vi "RandomLaser.vi"() -> ()   [LabVIEW 2014]
doc: "Random Laser Project\nAndré Romero - 2020\nandretec@ifsc.usp.br\n\nMain Program"
uses:
  OceanOptics.ctl
  PowerMeterSteps.ctl
  RL-Signal.ctl
  <vilib>/Analysis/2dsp.llb/Integral Method.ctl
  <vilib>/Analysis/8numeric.llb/1D Numeric Integration.vi
  GlobalVariables.vi
  <vilib>/Utility/file.llb/Write To Spreadsheet File (DBL).vi
  <vilib>/Analysis/NI_AAL_SigProc.lvlib
  <vilib>/Analysis/NI_AALBase.lvlib
  <vilib>/Analysis/NI_AALPro.lvlib
panel:
  in  "Stop":bool
  out "Power Meter":dbl[](array[numeric])=[-4.80034687e-05, -4.7408008e-05, -5.06443357e-05, -5.28425007e-05, -5.25678042e-05, -5.41400696e-05, -5.2216601e-05, -5.56666164e-05, -4.94078122e-05, -5.20333524e-05, -4.7408008e-05, -5.29950594e-05, -5.5727578e-05, -5.47354139e-05, -4.55456648e-05, -2.2403512e-05, -2.85706992e-05, -5.29950921e-05, -5.74067853e-05, -6.6779663e-05, -6.38182028e-05, -5.1773899e-05, -5.13617015e-05, -5.15602114e-05, -4.67210448e-05, -3.95311727e-05, -3.84473569e-05, -4.07676089e-05, -3.9119026e-05, -3.94700946e-05, -6.27801855e-05, -6.59400903e-05, -8.16175452e-05, -8.3525767e-05, -8.3525767e-05, -8.30677673e-05, -7.78622707e-05, -7.99309055e-06, 4.12680274e-05, 5.59075161e-05, 7.79505426e-05, 8.45298637e-05, 8.8880508e-05, 9.28800873e-05, 0.000106374602, 0.000115838942, 0.000191921004, 0.000232511724, 0.000233763392, 0.000173465407, 0.000158429335, 0.000152048175, 0.000145072074, 0.000134767964, 0.000126127823, 0.000116266419, 9.64061765e-05, 0.00010809963, 0.000134080954, 0.00013475267, 0.000128677129, 9.59789686e-05]
  out "Spectrum":dbl[][](array[numeric])
  out "Amplitudes":dbl[][](array[numeric])
  out "Locations Peaks":dbl[][](array[numeric])
  out "Integration":dbl[][](array[numeric])
  out "Integration":dbl[](array[numeric])
  out "size(s)":i32=105
  out "Waveform Graph 2":dbl[](graph)=[0.000604847446, 0.000604847446, 0.000604847446, 0.000688104541, 0.000688104541, 0.000688104541, 0.000688104541, 0.000915114302, 0.000915114302, 0.000915114302, 0.00125843158, 0.00125843158, 0.00125843158, 0.00169149181, 0.00169149181, 0.00169149181, 0.00169149181, 0.00235849386, 0.00235849386, 0.00235849386, 0.00235849386, 0.00314473268, 0.00314473268, 0.0041254824, 0.0041254824, 0.0041254824, 0.0041254824, 0.00483217463, 0.00483217463, 0.00483217463, 0.00559885986, 0.00559885986, 0.00559885986, 0.00559885986, 0.00666359905, 0.00666359905, 0.00666359905, 0.00792177953, 0.00792177953, 0.00792177953, 0.00792177953, 0.00900086574, 0.00900086574, 0.00900086574, 0.0102644078, 0.0102644078, 0.0102644078, 0.0102644078, 0.0114987111, 0.0114987111, 0.0114987111, 0.0114987111, 0.0129743796, 0.0129743796, 0.0129743796, 0.0141986832, 0.0141986832, 0.0141986832, 0.0141986832, 0.0155374203, 0.0155374203, 0.0155374203, 0.0155374203, 0.0168210845, 0.0168210845, 0.0168210845, 0.0182131026, 0.0182131026, 0.0182131026, 0.0182131026, 0.019541461, 0.019541461, 0.019541461, 0.0203341153, 0.0203341153, 0.0203341153, 0.0203341153, 0.0211376641, 0.0211376641, 0.0211376641, 0.0220639147, 0.0220639147, 0.0220639147, 0.0220639147, 0.0231049024, 0.0231049024, 0.0231049024, 0.0234890766, 0.0234890766, 0.0234890766, 0.0243229344, 0.0243229344, 0.0243229344, 0.0243229344, 0.0243483651, 0.0243483651, 0.0243483651, 0.0245883744, 0.0245883744, 0.0245883744, 0.0245883744, 0.0250559878, 0.0250559878, 0.0250559878, 0.0250559878]
  out "Motor Target":i32
  out "step error":dbl=5.243833813842798
  out "Numeric Control":i32=525
  out "appended array":dbl[](array[numeric])=[0.0239803754, 0.0238226056, 0.0238226056, 0.0238226056, 0.0243139379, 0.0243139379, 0.0243139379, 0.0243139379, 0.0240037385, 0.0240037385, 0.0240037385, 0.023470642, 0.023470642, 0.023470642, 0.0228483081, 0.0228483081, 0.0228483081, 0.0228483081, 0.0220416561, 0.0220416561, 0.0220416561, 0.0211109295, 0.0211109295, 0.0211109295, 0.0211109295, 0.0205111671, 0.0205111671, 0.0205111671, 0.0205111671, 0.0193525515, 0.0193525515, 0.0193525515, 0.0193525515, 0.0180644616, 0.0180644616, 0.0180644616, 0.0180644616, 0.0162604265, 0.0162604265, 0.0162604265, 0.0162604265, 0.015147699, 0.015147699, 0.0140616912, 0.0140616912, 0.0140616912, 0.0140616912, 0.0130754067, 0.0130754067, 0.0130754067, 0.0130754067, 0.0118028736, 0.0118028736, 0.0118028736, 0.0118028736, 0.00981818419, 0.00981818419, 0.00981818419, 0.00981818419, 0.00886647217, 0.00886647217, 0.00886647217, 0.00790723227, 0.00790723227, 0.00790723227, 0.00790723227, 0.00665996457, 0.00665996457, 0.00665996457, 0.00665996457, 0.00561416987, 0.00561416987, 0.00561416987, 0.00466312654, 0.00466312654, 0.00466312654, 0.00466312654, 0.00343694142, 0.00343694142, 0.00343694142, 0.00343694142, 0.00262781908, 0.00262781908, 0.00262781908, 0.00262781908, 0.00262781908, 0.0019172657, 0.0019172657, 0.0019172657, 0.0019172657, 0.0019172657, 0.00106541696, 0.00106541696, 0.00106541696, 0.00106541696, 0.000711521192, 0.000711521192, 0.000711521192, 0.000711521192, 0.000579979969, 0.000579979969, 0.000579979969, 0.000581125147, 0.000581125147, 0.000581125147, 0.000581125147, 0.000753699336, 0.000753699336, 0.000753699336, 0.000753699336, 0.00103271846, 0.00103271846, 0.00103271846, 0.00103271846, 0.00103271846, 0.00169448485, 0.00169448485, 0.00169448485, 0.00169448485, 0.00238372735, 0.00238372735, 0.00238372735, 0.00238372735, 0.00300710183, 0.00300710183, 0.00300710183, 0.00300710183, 0.00300710183, 0.00430094264, 0.00430094264, 0.00430094264, 0.00430094264, 0.00580574945, 0.00580574945, 0.00580574945, 0.00711680902, 0.00711680902, 0.00711680902, 0.00711680902, 0.0079354262, 0.0079354262, 0.0079354262, 0.0079354262, 0.00924165919, 0.00924165919, 0.00924165919, 0.0102110999, 0.0102110999, 0.0102110999, 0.0102110999, 0.0116844615, 0.0116844615, 0.0116844615, 0.0133227762, 0.0133227762, 0.0133227762, 0.0133227762, 0.0133227762, 0.0148326363, 0.0148326363, 0.0148326363, 0.0148326363, 0.0159355868, 0.0159355868, 0.0159355868, 0.0170806665, 0.0170806665, 0.0170806665, 0.0170806665, 0.0184924919, 0.0184924919, 0.0184924919, 0.0201629363, 0.0201629363, 0.0201629363, 0.0206157472, 0.0206157472, 0.0206157472, 0.0217395443, 0.0217395443, 0.0217395443, 0.0217395443, 0.0232210569, 0.0232210569, 0.0232210569, 0.023663858, 0.023663858, 0.023663858, 0.023663858, 0.023702329, 0.023702329, 0.023702329, 0.023702329, 0.0242230836, 0.0242230836, 0.0242230836, 0.0249410514, 0.0249410514, 0.0249410514, 0.0252798311, 0.0252798311, 0.0252798311, 0.0255696606, 0.0255696606, 0.0255696606, 0.0255696606, 0.0255696606, 0.025165854, 0.025165854, 0.025165854, 0.025165854, 0.0248792619, 0.0248792619, 0.0248792619, 0.0248792619, 0.0245558936, 0.0245558936, 0.0245558936, 0.0245558936, 0.024270013, 0.024270013, 0.024270013, 0.0235256515, 0.0235256515, 0.0235256515, 0.0235256515, 0.0228350237, 0.0228350237, 0.0228350237, 0.0228350237, 0.0225745663, 0.0225745663, 0.0225745663, 0.0225745663, 0.0210505258, 0.0210505258, 0.0210505258, 0.0210505258, 0.0199296717, 0.0199296717, 0.0199296717, 0.0199296717, 0.018528793, 0.018528793, 0.018528793, 0.018528793, 0.0175028276, 0.0175028276, 0.0175028276, 0.0158709381, 0.0158709381, 0.0158709381, 0.0158709381, 0.0138519667, 0.0138519667, 0.0138519667, 0.0131994681, 0.0131994681, 0.0131994681, 0.0131994681, 0.0117918346, 0.0117918346, 0.0117918346, 0.0107475519, 0.0107475519, 0.0107475519, 0.00919555873, 0.00919555873, 0.00919555873, 0.00919555873, 0.00811978336, 0.00811978336, 0.00811978336, 0.00811978336, 0.0069274581, 0.0069274581, 0.0069274581, 0.00582336541, 0.00582336541, 0.00582336541, 0.00582336541, 0.00476109795, 0.00476109795, 0.00476109795, 0.00476109795, 0.00476109795, 0.00366785936, 0.00366785936, 0.00366785936, 0.00366785936, 0.002746752, 0.002746752, 0.002746752, 0.002746752, 0.002746752, 0.00160831166, 0.00160831166, 0.00160831166, 0.0011865471, 0.0011865471, 0.0011865471, 0.0011865471, 0.00085388578, 0.00085388578, 0.00085388578, 0.00085388578, 0.0006647025, 0.0006647025, 0.0006647025, 0.000604847446, 0.000604847446, 0.000604847446, 0.000604847446, 0.000688104541, 0.000688104541, 0.000688104541, 0.000688104541, 0.000915114302, 0.000915114302, 0.000915114302, 0.00125843158, 0.00125843158, 0.00125843158, 0.00169149181, 0.00169149181, 0.00169149181, 0.00169149181, 0.00235849386, 0.00235849386, 0.00235849386, 0.00235849386, 0.00314473268, 0.00314473268, 0.0041254824, 0.0041254824, 0.0041254824, 0.0041254824, 0.00483217463, 0.00483217463, 0.00483217463, 0.00559885986, 0.00559885986, 0.00559885986, 0.00559885986, 0.00666359905, 0.00666359905, 0.00666359905, 0.00792177953, 0.00792177953, 0.00792177953, 0.00792177953, 0.00900086574, 0.00900086574, 0.00900086574, 0.0102644078, 0.0102644078, 0.0102644078, 0.0102644078, 0.0114987111, 0.0114987111, 0.0114987111, 0.0114987111, 0.0129743796, 0.0129743796, 0.0129743796, 0.0141986832, 0.0141986832, 0.0141986832, 0.0141986832, 0.0155374203, 0.0155374203, 0.0155374203, 0.0155374203, 0.0168210845, 0.0168210845, 0.0168210845, 0.0182131026, 0.0182131026, 0.0182131026, 0.0182131026, 0.019541461, 0.019541461, 0.019541461, 0.0203341153, 0.0203341153, 0.0203341153, 0.0203341153, 0.0211376641, 0.0211376641, 0.0211376641, 0.0220639147, 0.0220639147, 0.0220639147, 0.0220639147, 0.0231049024, 0.0231049024, 0.0231049024, 0.0234890766, 0.0234890766, 0.0234890766, 0.0243229344, 0.0243229344, 0.0243229344, 0.0243229344, 0.0243483651, 0.0243483651, 0.0243483651, 0.0245883744, 0.0245883744, 0.0245883744, 0.0245883744, 0.0250559878, 0.0250559878, 0.0250559878, 0.0250559878, 0.0253373459, 0.0253373459, 0.0253373459, 0.0249636527, 0.0249636527, 0.0249636527, 0.0249636527, 0.0249636527, 0.0248897653, 0.0248897653, 0.0248897653, 0.0244035777, 0.0244035777, 0.0244035777, 0.0244035777, 0.0237617642, 0.0237617642, 0.0237617642, 0.0237617642, 0.0230522826, 0.0230522826, 0.0230522826, 0.0230522826, 0.0222933218, 0.0222933218, 0.0222933218, 0.0222933218, 0.0213483702, 0.0213483702, 0.0213483702, 0.0213483702, 0.0201867707, 0.0201867707, 0.0201867707, 0.0201867707, 0.0201867707, 0.0185205508, 0.0185205508, 0.0185205508, 0.0185205508, 0.0185205508, 0.0163030662, 0.0163030662, 0.0163030662, 0.0151346121, 0.0151346121, 0.0151346121, 0.0151346121, 0.0136516355, 0.0136516355, 0.0136516355, 0.0136516355, 0.0121805826, 0.0121805826, 0.0121805826, 0.0121805826, 0.0110407537, 0.0110407537, 0.0110407537, 0.00959125254, 0.00959125254, 0.00959125254, 0.00959125254, 0.00959125254, 0.00828862097, 0.00828862097, 0.00828862097, 0.00828862097, 0.00685082562, 0.00685082562, 0.00685082562, 0.00575551065, 0.00575551065, 0.00575551065, 0.00575551065, 0.00451412285, 0.00451412285, 0.00451412285, 0.00335313403, 0.00335313403, 0.00335313403, 0.00267822552, 0.00267822552, 0.00267822552, 0.00267822552, 0.00208994723, 0.00208994723, 0.00208994723, 0.00208994723, 0.00154257915, 0.00154257915, 0.00154257915, 0.00107440748, 0.00107440748, 0.00107440748, 0.00107440748, 0.00079549622, 0.00079549622, 0.00079549622, 0.00079549622, 0.00079549622, 0.000625455519, 0.000625455519, 0.000625455519, 0.000625455519, 0.000673602568, 0.000673602568, 0.000673602568, 0.000673602568, 0.000673602568, 0.000927159155]
  out "Locations":dbl[](array[numeric])=[101.70035202549552, 310.107546258005, 519.7561661861572]
  out "Amplitudes":dbl[](array[numeric])=[0.000558557811238861, 0.000615890857834203, 0.0006343968853356121]
  out "standard deviation":dbl=0.877820527728183 format="%0.2f"
  out "mean":dbl=209.02790708033083 format="%0.2f"
  out "Array":dbl[](array[numeric])=[208.40719423250948, 209.6486199281522]
  out "# found":i32=3
  in  "Select Light Source":u16(ring)=6
  in  "Tab Control":T1(tab)=enum."Aquisition"
  out "Current Position":dbl=62.0
  out "Min power to Aqc":dbl
  out "Max power to Aqc":dbl
  out "Low power":bool
  out "Max power":bool
  in  "Clear Dark Spec":bool caption="Blank Button"
  in  "Average":i32=1
  in  "Integration Time":i32=100
  out "Spectrum":T2(graph)
  in  "Store Dark Spec":bool caption="Blank Button"
  out "table":string[][](table)=[["nm", "Peak"]]
  in  "threshold":dbl=5000.0 format="%0.2f"
  in  "width":i32=10 min=3
  out "Power Meter [W]":dbl=-6.24901586e-05 format="%#_4p"
  in  "Power up":bool
  in  "Power down":bool
  in  "Half Power":bool
  in  "min Power":bool
  in  "max Power Go":bool
  out "Max Power":dbl=0.0255696606 format="%#_3p"
  out "Min Power":dbl=0.000579979969 format="%#_3p"
  in  "Correct Electrical Dark":bool
  out "Power Meter":dbl=-6.24901586e-05 format="%#_4p"
  in  "Tuning Motor":bool
  out "Power Meter":dbl(graph)=0.000927159155
  out "Min Power":dbl=0.000579979969 format="%#_3p"
  out "Max Power":dbl=0.0255696606 format="%#_3p"
  out "Power Meter [W]":dbl=-6.24901586e-05 format="%#_4p"
  out "Running":bool
  out "Amostra":cluster{dbl[], dbl[]}(graph)={[-4.80034687e-05, -4.7408008e-05, -5.06443357e-05, -5.28425007e-05, -5.25678042e-05, -5.41400696e-05, -5.2216601e-05, -5.56666164e-05, -4.94078122e-05, -5.20333524e-05, -4.7408008e-05, -5.29950594e-05, -5.5727578e-05, -5.47354139e-05, -4.55456648e-05, -2.2403512e-05, -2.85706992e-05, -5.29950921e-05, -5.74067853e-05, -6.6779663e-05, -6.38182028e-05, -5.1773899e-05, -5.13617015e-05, -5.15602114e-05, -4.67210448e-05, -3.95311727e-05, -3.84473569e-05, -4.07676089e-05, -3.9119026e-05, -3.94700946e-05, -6.27801855e-05, -6.59400903e-05, -8.16175452e-05, -8.3525767e-05, -8.3525767e-05, -8.30677673e-05, -7.78622707e-05, -7.99309055e-06, 4.12680274e-05, 5.59075161e-05, 7.79505426e-05, 8.45298637e-05, 8.8880508e-05, 9.28800873e-05, 0.000106374602, 0.000115838942, 0.000191921004, 0.000232511724, 0.000233763392, 0.000173465407, 0.000158429335, 0.000152048175, 0.000145072074, 0.000134767964, 0.000126127823, 0.000116266419, 9.64061765e-05, 0.00010809963, 0.000134080954, 0.00013475267, 0.000128677129, 9.59789686e-05], []}
  in  "Step Stop":i32=105
  in  "Save Aquisition":bool
  in  "Play Aquisition":bool
  out "Laser":cluster{dbl[], dbl[]}(graph)={[-4.80034687e-05, -4.7408008e-05, -5.06443357e-05, -5.28425007e-05, -5.25678042e-05, -5.41400696e-05, -5.2216601e-05, -5.56666164e-05, -4.94078122e-05, -5.20333524e-05, -4.7408008e-05, -5.29950594e-05, -5.5727578e-05, -5.47354139e-05, -4.55456648e-05, -2.2403512e-05, -2.85706992e-05, -5.29950921e-05, -5.74067853e-05, -6.6779663e-05, -6.38182028e-05, -5.1773899e-05, -5.13617015e-05, -5.15602114e-05, -4.67210448e-05, -3.95311727e-05, -3.84473569e-05, -4.07676089e-05, -3.9119026e-05, -3.94700946e-05, -6.27801855e-05, -6.59400903e-05, -8.16175452e-05, -8.3525767e-05, -8.3525767e-05, -8.30677673e-05, -7.78622707e-05, -7.99309055e-06, 4.12680274e-05, 5.59075161e-05, 7.79505426e-05, 8.45298637e-05, 8.8880508e-05, 9.28800873e-05, 0.000106374602, 0.000115838942, 0.000191921004, 0.000232511724, 0.000233763392, 0.000173465407, 0.000158429335, 0.000152048175, 0.000145072074, 0.000134767964, 0.000126127823, 0.000116266419, 9.64061765e-05, 0.00010809963, 0.000134080954, 0.00013475267, 0.000128677129, 9.59789686e-05], []}
  out "Power Value":dbl=-6.24901586e-05 caption="Optical Power [W]" format="%#_4p"
  in  "Average Time (0.0)":dbl=0.05
  out "P Meter Delay (ms)":u32=203
  out "Spectrum delay (ms)":u32=300
  # "Set power to Aquisition"
  # "Move Step Motor"
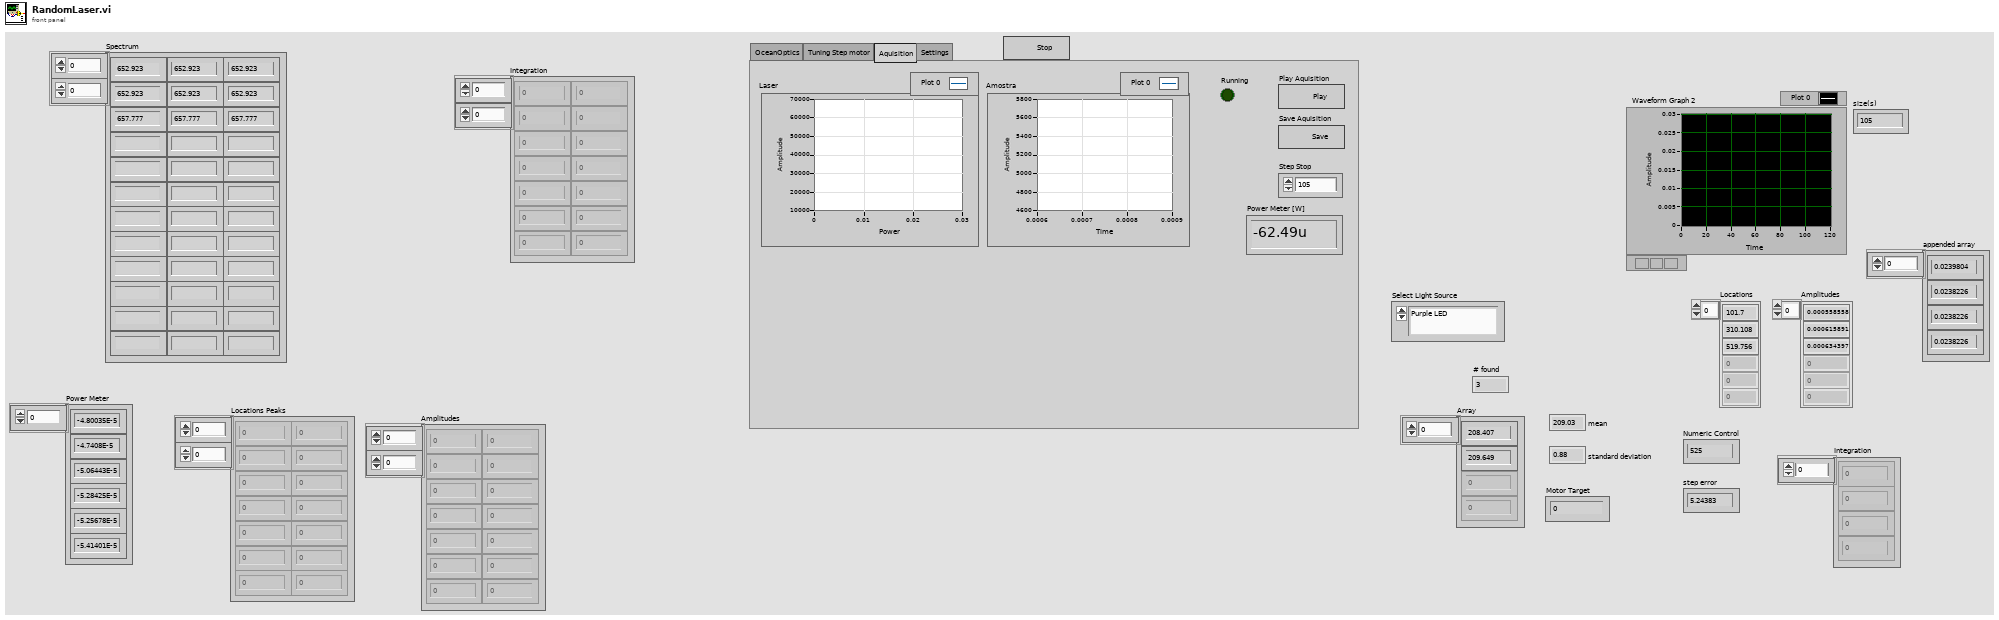
[diagram p1: front panel]
types:
  T1 = enum32{"OceanOptics", "Tuning Step motor", "Aquisition", "Settings"}
  T2 = cluster{"WL Values":dbl[], "Spectrum Values":dbl[]}[]
  T3 = typedef "PowerMeterSteps.ctl" = enum16{"Initialize", "Graph", "Wait for Event", "Tuning", "Get Power", "MoveMotor", "corrects step"}
  T4 = typedef "OceanOptics.ctl" = enum16{"Initialize", "Graph", "Wait for Event", "Dark Spec", "Clear Dark Spec", "OceanOptics", "Create File", "Save"}
  T5 = enum16{"open", "replace", "create", "open or create", "replace or create", "replace or create with confirmation"}
  T6 = typedef "RL-Signal.ctl" = cluster{"Signal State":string, "Step":dbl, "Spectrum":dbl[][], "Amplitudes":dbl[], "Locations":dbl[], "Integration":dbl[], "Error":errorcluster}
  T7 = cluster{"WL Values":dbl[], "Spectrum Values":dbl[]}
  T8 = cluster{"Wavelenght":dbl[], "Spectrum Values":dbl[]}
  T9 = typedef "NI_AALPro.lvlib/Integral Method.ctl" = i32
  T10 = cluster{"Locations WL":dbl[], "Amplitudes":dbl[]}
  T11 = cluster{"Locations WL":dbl[], "Amplitudes":dbl[]}[]
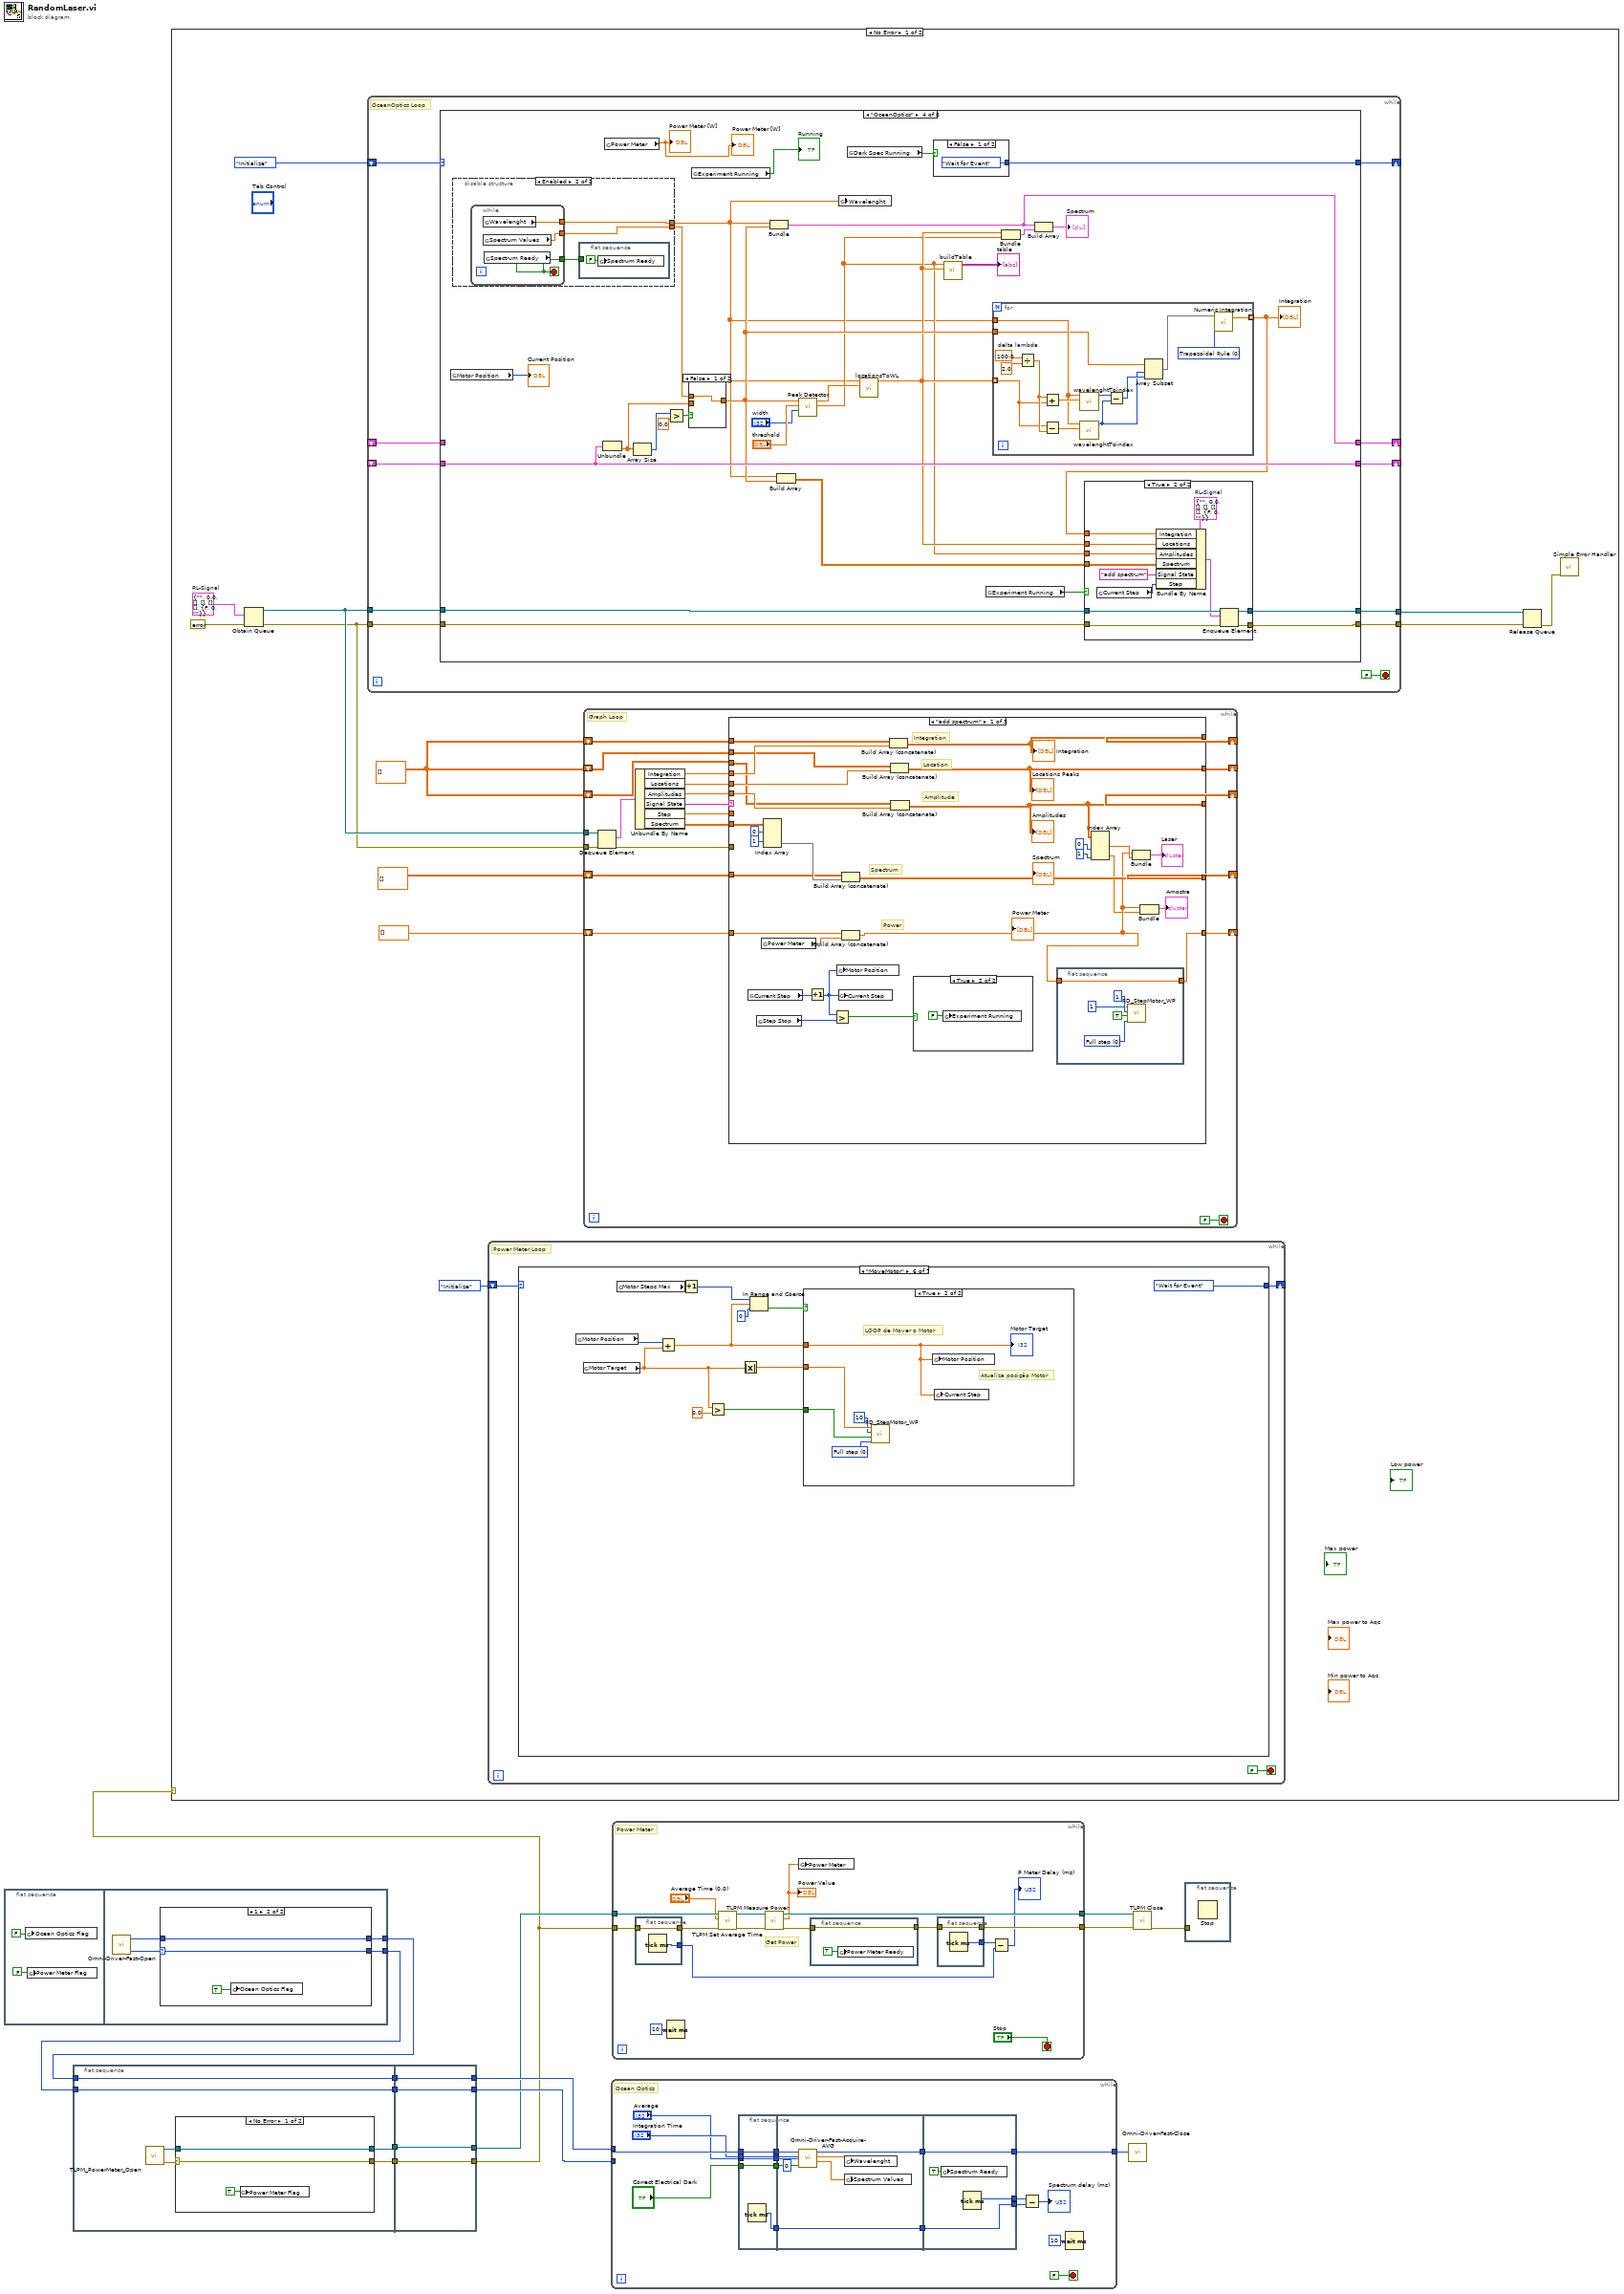
[diagram p0: block diagram]
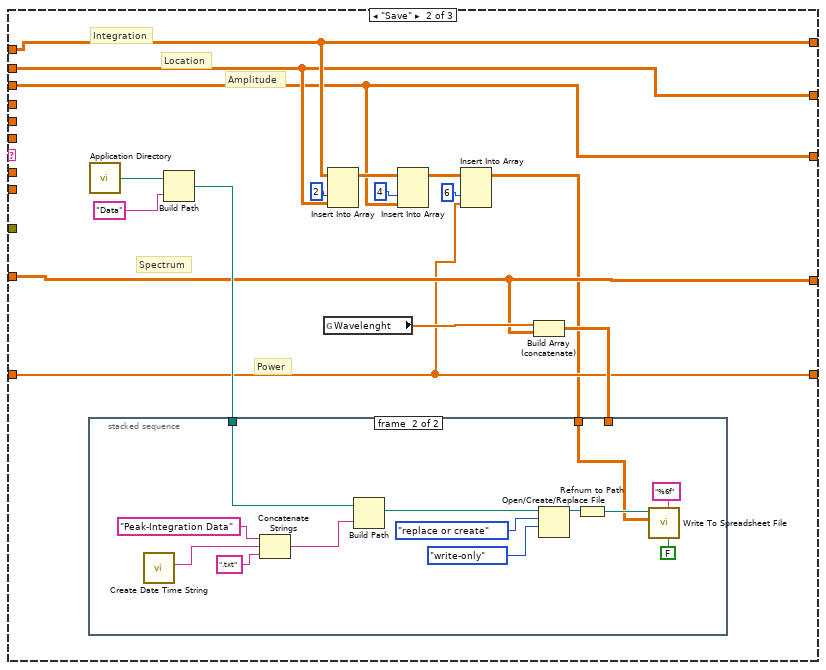
[diagram p3: hidden frame]
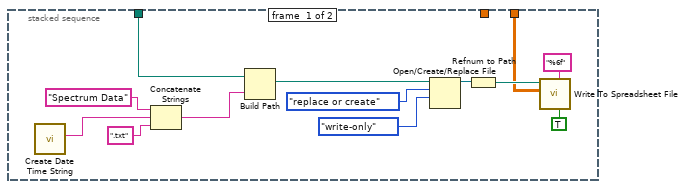
[diagram p4: hidden frame]
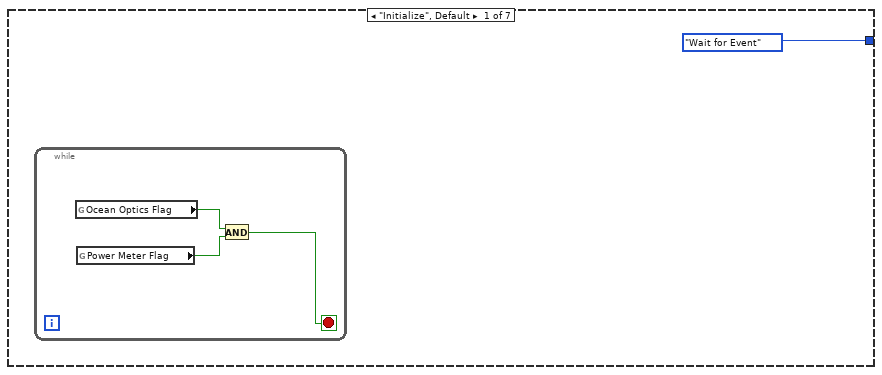
[diagram p6: hidden frame]
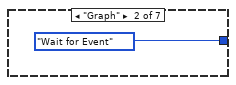
[diagram p7: hidden frame]
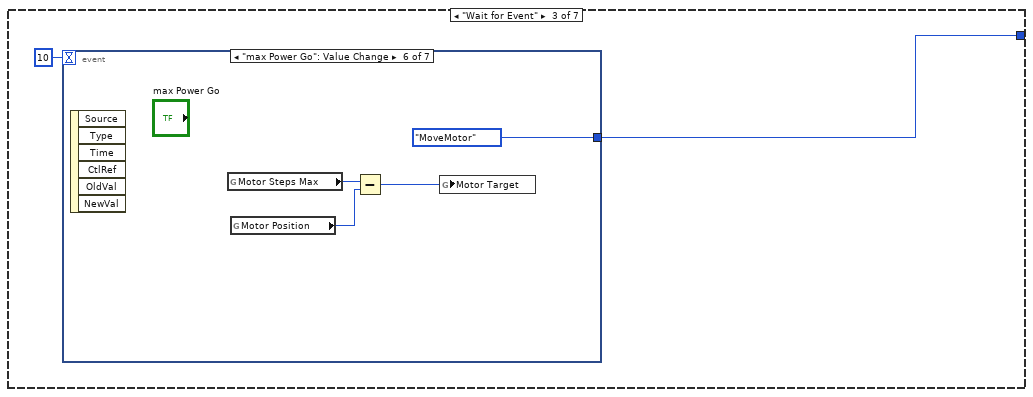
[diagram p8: hidden frame]
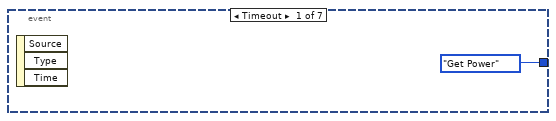
[diagram p9: hidden frame]
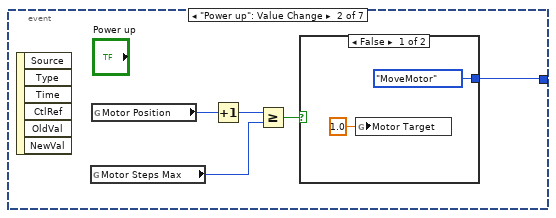
[diagram p10: hidden frame]
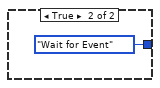
[diagram p11: hidden frame]
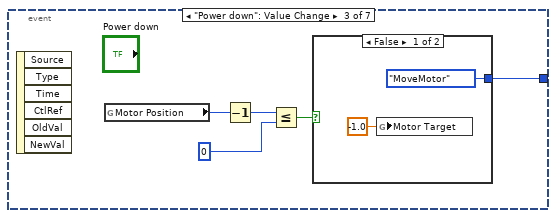
[diagram p12: hidden frame]
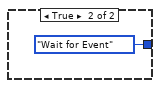
[diagram p13: hidden frame]
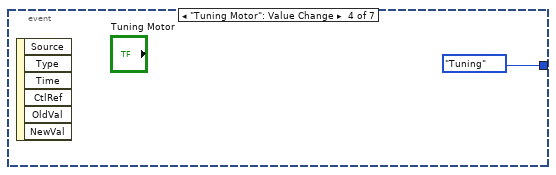
[diagram p14: hidden frame]
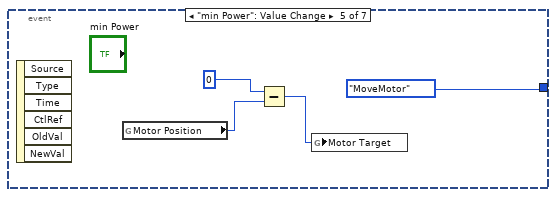
[diagram p15: hidden frame]
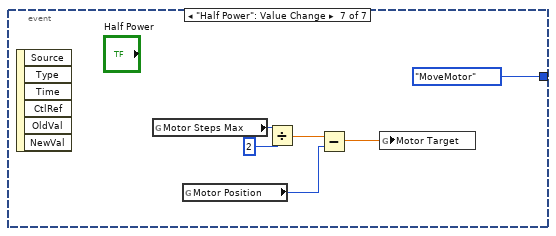
[diagram p16: hidden frame]
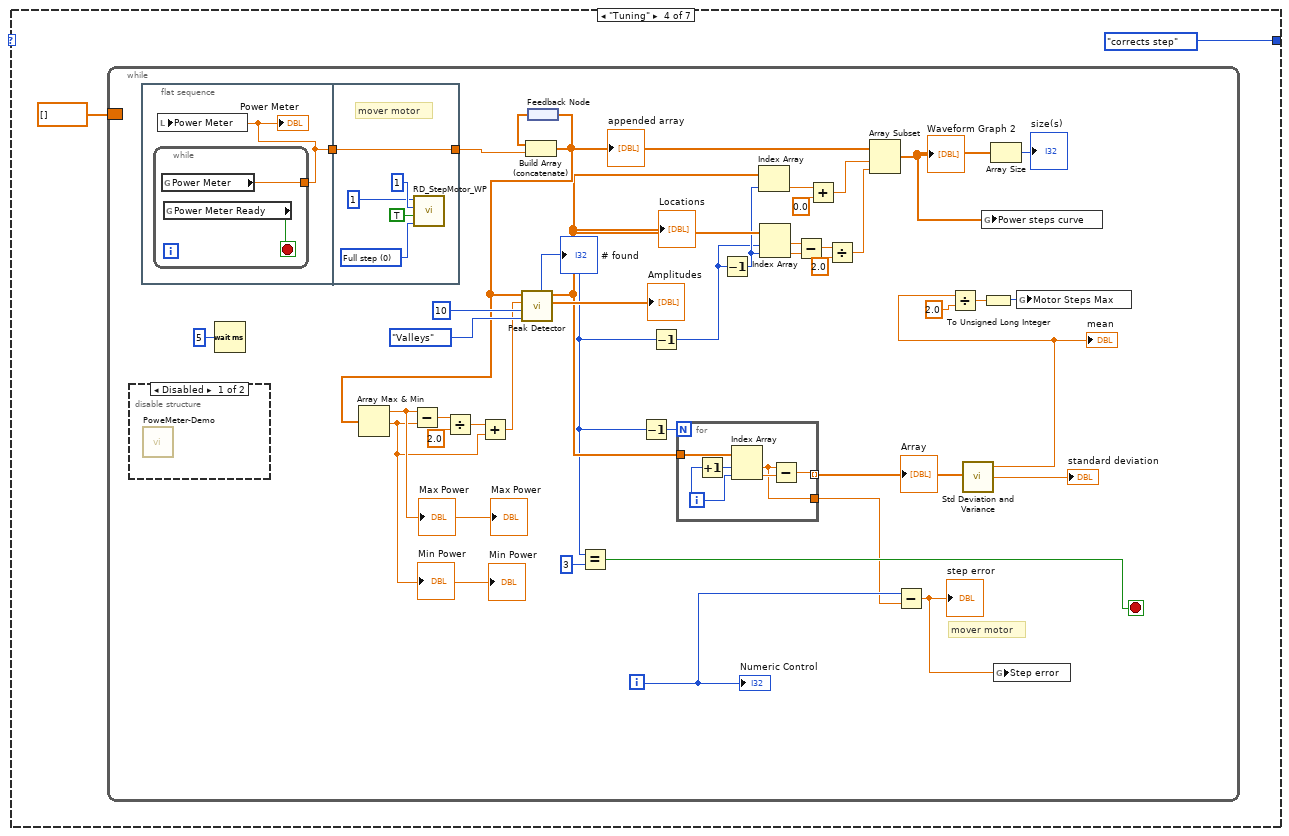
[diagram p17: hidden frame]
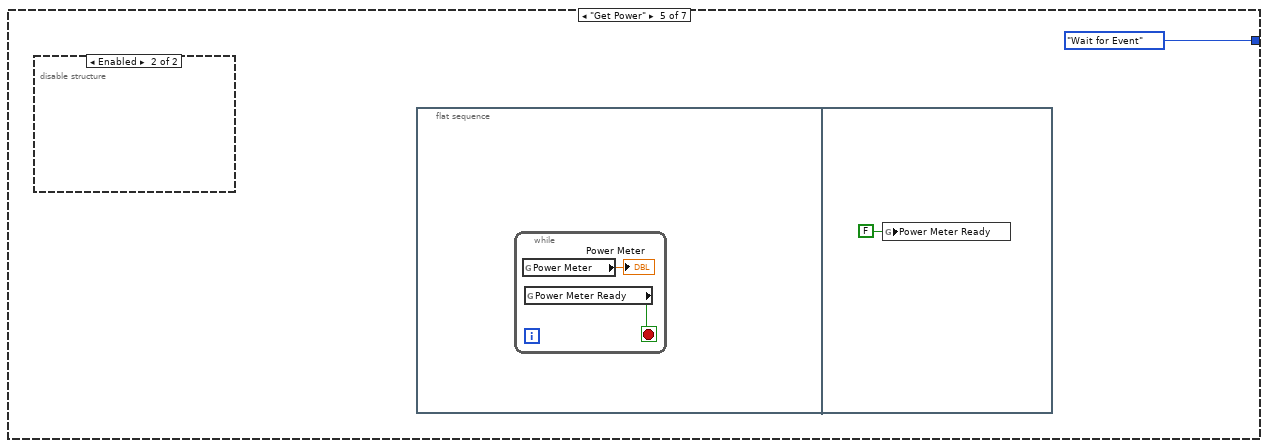
[diagram p19: hidden frame]
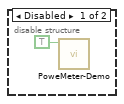
[diagram p20: hidden frame]
diagram:
  n1 = flat-sequence {
    tunnel: [w18] -> w8
    tunnel: [w17] -> w7
    frame #0 {
      n2 = global write "GlobalVariables.vi" "Ocean Optics Flag"(FALSE ("Ocean Optics")) -> ()
      n3 = global write "GlobalVariables.vi" "Power Meter Flag"(FALSE ("Ocean Optics")) -> ()
    }
    frame #1 {
      n4 = call "Omni-Driver-Fast-Open.vi"() -> ("Number of Spectrometers"=w20:i32, "Wrapper Out"=w19:u32)  [unwired: 4 in]
      n5 = case shown="1" w20 {
        selector: w20 -> [_ w23]
        tunnel: w19 -> [_ w24]
        tunnel: [_ w24] -> w18
        tunnel: [_ w23] -> w17
        frame 0, Default {
          n6 = flat-sequence {
            frame #0 {
              n7 = One Button Dialog(message="Ocean Optics not Connected") -> ()  [unwired: 1 in, 1 out]
            }
            frame #1 {
              n8 = Stop() -> ()  [unwired: 1 in]
            }
          }
        }
        frame 1 {
          n9 = global write "GlobalVariables.vi" "Ocean Optics Flag"(TRUE ("Ocean Optics")) -> ()
        }
      }
    }
  }
  n10 = flat-sequence {
    tunnel: [w28] -> w10
    tunnel: [w27] -> w9
    tunnel: w8 -> [w26]
    tunnel: w7 -> [w25]
    tunnel: [w26] -> w6
    tunnel: [w25] -> w3
    tunnel: w10 -> [w38]
    tunnel: [w38] -> w2
    tunnel: [w37] -> w1
    tunnel: w9 -> [w37]
    tunnel: [w36] -> w5
    tunnel: w6 -> [w36]
    tunnel: [w35] -> w4
    tunnel: w3 -> [w35]
    frame #0 {
      n11 = call "TLPM_PowerMeter_Open.vi"() -> ("error out"=w30:errorcluster, "instrument handle out"=w29:refnum<visa-resource-name>)  [unwired: 10 in]
      n12 = case shown="No Error" w30 {
        selector: w30 -> [w32 _]
        tunnel: w29 -> [w33 _]
        tunnel: [w33 _] -> w28
        tunnel: [w32 _] -> w27
        frame No Error {
          n13 = global write "GlobalVariables.vi" "Power Meter Flag"(TRUE ("Ocean Optics")) -> ()
        }
        frame Error {
          n14 = flat-sequence {
            frame #0 {
              n15 = One Button Dialog(message="Power Meter not Connected") -> ()  [unwired: 1 in, 1 out]
            }
            frame #1 {
              n16 = Stop() -> ()  [unwired: 1 in]
            }
          }
        }
      }
    }
    frame #1 {
    }
  }
  n17 = case shown="No Error" w1 {
    frame No Error {
      w43 = dbl[][] []
      w47 = T6 {"Signal State"="", "Step"=0.0, "Spectrum"=[], "Amplitudes"=[], "Locations"=[], "Integration"=[], "Error"={"status"=FALSE, "code"=0, "source"=""}}  # RL-Signal
      n18 = Obtain Queue(element data type=w47, error in (no error)=errorcluster {"status"=FALSE, "code"=0, "source"=""}) -> (queue out=w46:refnum<queue>, error out=w45:errorcluster)  [unwired: 3 in, 1 out]
      n19 = while {
        shift-right: [w286] -> _
        shift-left: OceanOptics."Initialize" -> [w283]
        shift-right: [w289] -> _
        shift-left: _ -> [w288]
        shift-right: [w285] -> _
        shift-left: _ -> [w284]
        tunnel: w45 -> [w282]
        tunnel: w46 -> [w281]
        tunnel: [w280] -> w40
        tunnel: [w279] -> w39
        stop <- FALSE stop-if-true
        # "OceanOptics Loop"
        n20 = case shown="\"OceanOptics\"" w283 {
          tunnel: [w293 w302 w308 w333 w394 w399 w401 w411] -> w289
          tunnel: w288 -> [_ w302 w308 _ w394 w399 w401 w411]
          tunnel: [OceanOptics."OceanOptics" OceanOptics."OceanOptics" w307 w339 OceanOptics."OceanOptics" OceanOptics."OceanOptics" OceanOptics."OceanOptics" OceanOptics."OceanOptics"] -> w286
          tunnel: [w293 w302 w305 w345 w393 w398 w400 w410] -> w285
          tunnel: w284 -> [_ _ w305 w345 w393 _ w400 w410]
          tunnel: w282 -> [w291 w298 w303 w328 w390 w395 _ w414]
          tunnel: w281 -> [w292 w299 w304 w329 w391 w396 w407 w415]
          tunnel: [w292 w299 w304 w325 w391 w396 w404 w413] -> w280
          tunnel: [w291 w298 w303 w324 w390 w395 w403 w412] -> w279
          frame "Initialize", Default {
            w290 = 0 ("Motor Position")
            w293 = T7 {"WL Values"=[], "Spectrum Values"=[]}  # clear graph
            n21 = while {
              stop <- w295 stop-if-true
              n22 = global read "GlobalVariables.vi" "Ocean Optics Flag"() -> (w297:bool)
              n23 = global read "GlobalVariables.vi" "Power Meter Flag"() -> (w296:bool)
              n24 = And(x=w297, y=w296) -> (x .and. y?=w295:bool)
            }
            n25 = global write "GlobalVariables.vi" "Motor Position"(w290) -> ()
            n26 = global write "GlobalVariables.vi" "Current Step"(w290) -> ()
          }
          frame "Dark Spec" {
            n27 = global write "GlobalVariables.vi" "Dark Spec Running"(FALSE ("Dark Spec Running")) -> ()
          }
          frame "Wait for Event" {
            n28 = event shown="[2] \"Play Aquisition\": Value Change" {
              selector: _ -> [_ _ _ _ _]
              dyn-events: _ -> [_ _ _ _ _]
              timeout: 10 -> [_ _ _ _ _]
              tunnel: [OceanOptics."OceanOptics" OceanOptics."Clear Dark Spec" OceanOptics."OceanOptics" OceanOptics."Save" OceanOptics."Clear Dark Spec"] -> w307
              event Timeout {
                n29 = event-data() -> ()  [unwired: 1 in, 3 out]
              }
              event "Store Dark Spec": Value Change {
                n30 = event-data() -> ()  [unwired: 1 in, 3 out]
                n31 = global write "GlobalVariables.vi" "Dark Spec Running"(TRUE ("Dark Spec Running")) -> ()
              }
              event "Play Aquisition": Value Change {
                n32 = event-data() -> ()  [unwired: 1 in, 3 out]
                n33 = global write "GlobalVariables.vi" "Experiment Running"(TRUE ("Experiment Running")) -> ()
                n34 = global write "GlobalVariables.vi" "Step Stop"("Step Stop") -> ()
              }
              event "Save Aquisition": Value Change {
                n35 = event-data() -> ()  [unwired: 1 in, 3 out]
              }
              event "Clear Dark Spec": Value Change {
                n36 = event-data() -> ()  [unwired: 1 in, 3 out]
              }
            }
          }
          frame "OceanOptics" {
            n37 = global read "GlobalVariables.vi" "Motor Position"() -> (→"Current Position":i32)
            n38 = disable-structure shown="Enabled" {
              disable-tunnel: [w348 w350] -> w341
              disable-tunnel: [w346 w351] -> w320
              frame Disabled {
                n39 = call "SpectrumOfLight.vi"("Select Light Source"="Select Light Source") -> ("Spectrum Values"=w348:dbl[], "WL Values"=w346:dbl[])  [unwired: 9 in]
              }
              frame Enabled {
                n40 = while {
                  tunnel: [w355] -> w351
                  tunnel: [w354] -> w350
                  tunnel: [w353] -> w349
                  stop <- w353 stop-if-true
                  n41 = global read "GlobalVariables.vi" "Wavelenght"() -> (w355:dbl[])
                  n42 = global read "GlobalVariables.vi" "Spectrum Values"() -> (w354:dbl[])
                  n43 = global read "GlobalVariables.vi" "Spectrum Ready"() -> (w353:bool)
                }
                n44 = flat-sequence {
                  tunnel: w349 -> [_]
                  frame #0 {
                    n45 = global write "GlobalVariables.vi" "Spectrum Ready"(FALSE ("Spectrum Ready")) -> ()
                  }
                }
              }
            }
            n46 = Unbundle(w345) -> ("Spectrum Values"=w340:dbl[])  [unwired: 1 out]
            n47 = global read "GlobalVariables.vi" "Power Meter"() -> (→"Power Meter [W]" →"Power Meter [W]":dbl)
            n48 = Array Size(array=w340) -> (size(s)=w342:i32)
            n49 = Greater?(x=w342, y=0.0) -> (0:w344:bool)
            n50 = case shown="False" w344 {
              tunnel: w341 -> [w386 w389]
              tunnel: w340 -> [_ w388]
              tunnel: [w386 w387] -> w327
              frame False {
              }
              frame True {
                n51 = Subtract(x=w389, y=w388) -> (x-y=w387:dbl[])
              }
            }
            n52 = global read "GlobalVariables.vi" "Experiment Running"() -> (→"Running":bool)
            n53 = Bundle("Wavelenght"=w320, "Spectrum Values"=w327) -> (w333:T8)  [unwired: 1 in]
            n54 = Build Array(w320, w327) -> (w326:dbl[][])
            n55 = call <vilib>:"Peak Detector.vi"("width"="width", "threshold"="threshold", "X"=w327) -> ("Amplitudes"=w321:dbl[], "Locations"=w335:dbl[])  [unwired: 4 in, 3 out]
            n56 = global write "GlobalVariables.vi" "Wavelenght"(w320) -> ()
            n57 = global read "GlobalVariables.vi" "Dark Spec Running"() -> (w338:bool)
            n58 = call "locationsToWL.vi"("Locations index"=w335, "WL Values"=w320) -> ("Locations WL"=w322:dbl[])  [unwired: 9 in]
            n59 = case shown="False" w338 {
              tunnel: [OceanOptics."Wait for Event" OceanOptics."Dark Spec"] -> w339
              frame False {
              }
              frame True {
              }
            }
            n60 = call "buildTable.vi"("Locations"=w322, "Amplitudes"=w321) -> ("Table"=→"table":string[][])  [unwired: 9 in]
            n61 = global read "GlobalVariables.vi" "Experiment Running"() -> (w330:bool)
            n62 = for {
              tunnel: w322 -> [w380] mode=indexing
              tunnel: w320 -> [w377]
              tunnel: w327 -> [w375]
              tunnel: [w371] -> w323 mode=indexing
              w372 = T9 0 items=["Trapezoidal Rule", "Simpson's Rule", "Simpson's 3/8 Rule", "Bode Rule"] ("integration method")
              w383 = 100.0  # delta lambda
              n63 = Divide(x=w383, y=2.0) -> (x/y=w381:dbl)
              n64 = Add(x=w381, y=w380) -> (x+y=w379:dbl)
              n65 = Subtract(x=w380, y=w381) -> (x-y=w378:dbl)
              n66 = call "wavelenghtToindex.vi"("WL in"=w379, "WL Values"=w377) -> ("index of WL"=w376:i32)  [unwired: 9 in]
              n67 = call "wavelenghtToindex.vi"("WL in"=w378, "WL Values"=w377) -> ("index of WL"=w373:i32)  [unwired: 9 in]
              n68 = Subtract(x=w376, y=w373) -> (x-y=w374:i32)
              n69 = Array Subset(array=w375, index=w373, length=w374) -> (w370:dbl[])
              n70 = call-poly <vilib>:"Numeric Integration.vi"("integration method"=w372, "Input Array"=w370) -> ("result"=w371:dbl)  [unwired: 1 in, 1 out]
            }
            "Integration" <- w323
            n71 = Bundle("Locations WL"=w322, "Amplitudes"=w321) -> (w334:T10)  [unwired: 1 in]
            n72 = Build Array(w333, w334) -> (→"Spectrum":T11)
            n73 = case shown="True" w330 {
              tunnel: w329 -> [w357 w367]
              tunnel: w328 -> [w356 w366]
              tunnel: w326 -> [_ w364]
              tunnel: [w357 w363] -> w325
              tunnel: [w356 w362] -> w324
              tunnel: w323 -> [_ w360]
              tunnel: w322 -> [_ w359]
              tunnel: w321 -> [_ w358]
              frame False {
              }
              frame True {
                w369 = T6 {"Signal State"="", "Step"=0.0, "Spectrum"=[], "Amplitudes"=[], "Locations"=[], "Integration"=[], "Error"={"status"=FALSE, "code"=0, "source"=""}}  # RL-Signal
                n74 = global read "GlobalVariables.vi" "Current Step"() -> (w361:i32)
                n75 = Bundle By Name(cluster=w369, "Integration"=w360, "Locations"=w359, "Amplitudes"=w358, "Spectrum"=w364, "Signal State"="add spectrum", "Step"=w361) -> (w365:T6)
                n76 = Enqueue Element(queue=w367, element=w365, error in (no error)=w366) -> (queue out=w363:refnum<queue>, error out=w362:errorcluster)  [unwired: 1 in, 1 out]
              }
            }
          }
          frame "Graph" {
          }
          frame "Clear Dark Spec" {
            w398 = T7 {"WL Values"=[], "Spectrum Values"=[]}  # clear graph
          }
          frame "Create File" {
            w406 = T6 {"Signal State"="", "Step"=0.0, "Spectrum"=[], "Amplitudes"=[], "Locations"=[], "Integration"=[], "Error"={"status"=FALSE, "code"=0, "source"=""}}  # RL-Signal
            n77 = Bundle By Name(cluster=w406, "Signal State"="Create File") -> (w405:T6)
            n78 = Enqueue Element(queue=w407, element=w405) -> (queue out=w404:refnum<queue>, error out=w403:errorcluster)  [unwired: 2 in, 1 out]
          }
          frame "Save" {
            w417 = T6 {"Signal State"="", "Step"=0.0, "Spectrum"=[], "Amplitudes"=[], "Locations"=[], "Integration"=[], "Error"={"status"=FALSE, "code"=0, "source"=""}}  # RL-Signal
            n79 = Bundle By Name(cluster=w417, "Signal State"="Save") -> (w416:T6)
            n80 = Enqueue Element(queue=w415, element=w416, error in (no error)=w414) -> (queue out=w413:refnum<queue>, error out=w412:errorcluster)  [unwired: 1 in, 1 out]
          }
        }
      }
      n81 = while {
        shift-right: [w154] -> _
        shift-left: PowerMeterSteps."Initialize" ("Enum") -> [w155]
        stop <- FALSE stop-if-true
        # "Power Meter Loop"
        n82 = case shown="\"MoveMotor\"" w155 {
          tunnel: [PowerMeterSteps."Wait for Event" ("Enum") PowerMeterSteps."Wait for Event" ("Enum") w163 PowerMeterSteps."corrects step" ("Enum") PowerMeterSteps."Wait for Event" ("Enum") PowerMeterSteps."Wait for Event" ("Enum") PowerMeterSteps."Wait for Event" ("Enum")] -> w154
          frame "Initialize", Default {
            n83 = while {
              stop <- w158 stop-if-true
              n84 = global read "GlobalVariables.vi" "Ocean Optics Flag"() -> (w160:bool)
              n85 = global read "GlobalVariables.vi" "Power Meter Flag"() -> (w159:bool)
              n86 = And(x=w160, y=w159) -> (x .and. y?=w158:bool)
            }
          }
          frame "Graph" {
          }
          frame "Wait for Event" {
            n87 = event shown="[5] \"max Power Go\": Value Change" {
              selector: _ -> [_ _ _ _ _ _ _]
              dyn-events: _ -> [_ _ _ _ _ _ _]
              timeout: 10 -> [_ _ _ _ _ _ _]
              tunnel: [PowerMeterSteps."Get Power" ("Enum") w166 w173 PowerMeterSteps."Tuning" ("Enum") PowerMeterSteps."MoveMotor" ("Enum") PowerMeterSteps."MoveMotor" ("Enum") PowerMeterSteps."MoveMotor" ("Enum")] -> w163
              event Timeout {
                n88 = event-data() -> ()  [unwired: 1 in, 3 out]
              }
              event "Power up": Value Change {
                n89 = event-data() -> ()  [unwired: 1 in, 6 out]
                n90 = global read "GlobalVariables.vi" "Motor Steps Max"() -> (w168:i32)
                n91 = global read "GlobalVariables.vi" "Motor Position"() -> (w169:i32)
                n92 = Increment(x=w169) -> (x+1=w165:i32)
                n93 = Greater Or Equal?(x=w165, y=w168) -> (x >= y?=w167:bool)
                n94 = case shown="False" w167 {
                  tunnel: [PowerMeterSteps."MoveMotor" ("Enum") PowerMeterSteps."Wait for Event" ("Enum")] -> w166
                  frame False {
                    n95 = global write "GlobalVariables.vi" "Motor Target"(1.0 ("Motor Target")) -> ()
                  }
                  frame True {
                  }
                }
              }
              event "Power down": Value Change {
                n96 = event-data() -> ()  [unwired: 1 in, 6 out]
                n97 = global read "GlobalVariables.vi" "Motor Position"() -> (w175:i32)
                n98 = Decrement(x=w175) -> (x-1=w177:i32)
                n99 = Less Or Equal?(x=w177, y=0) -> (x <= y?=w176:bool)
                n100 = case shown="False" w176 {
                  tunnel: [PowerMeterSteps."MoveMotor" ("Enum") PowerMeterSteps."Wait for Event" ("Enum")] -> w173
                  frame False {
                    n101 = global write "GlobalVariables.vi" "Motor Target"(-1.0 ("Motor Target")) -> ()
                  }
                  frame True {
                  }
                }
              }
              event "Tuning Motor": Value Change {
                n102 = event-data() -> ()  [unwired: 1 in, 6 out]
              }
              event "min Power": Value Change {
                n103 = event-data() -> ()  [unwired: 1 in, 6 out]
                n104 = global read "GlobalVariables.vi" "Motor Position"() -> (w183:i32)
                n105 = Subtract(x=0, y=w183) -> (x-y=w182:i32)
                n106 = global write "GlobalVariables.vi" "Motor Target"(w182) -> ()
              }
              event "max Power Go": Value Change {
                n107 = event-data() -> ()  [unwired: 1 in, 6 out]
                n108 = global read "GlobalVariables.vi" "Motor Steps Max"() -> (w188:i32)
                n109 = global read "GlobalVariables.vi" "Motor Position"() -> (w187:i32)
                n110 = Subtract(x=w188, y=w187) -> (x-y=w186:i32)
                n111 = global write "GlobalVariables.vi" "Motor Target"(w186) -> ()
              }
              event "Half Power": Value Change {
                n112 = event-data() -> ()  [unwired: 1 in, 6 out]
                n113 = global read "GlobalVariables.vi" "Motor Steps Max"() -> (w194:i32)
                n114 = global read "GlobalVariables.vi" "Motor Position"() -> (w191:i32)
                n115 = Divide(x=w194, y=2) -> (x/y=w192:dbl)
                n116 = Subtract(x=w192, y=w191) -> (x-y=w190:dbl)
                n117 = global write "GlobalVariables.vi" "Motor Target"(w190) -> ()
              }
            }
          }
          frame "Tuning" {
            n118 = while {
              border: dbl[] [] -> [_]
              i -> [w223]
              stop <- w226 stop-if-true
              # "mover motor"
              n119 = disable-structure shown="Disabled" {
                frame Disabled {
                  n120 = call "PoweMeter-Demo.vi"() -> ()  [unwired: 10 in, 2 out]
                }
                frame Enabled {
                }
              }
              n121 = flat-sequence {
                tunnel: [w238] -> w216
                tunnel: [w245] -> w217
                tunnel: w216 -> [w245]
                frame #0 {
                  n122 = while {
                    tunnel: [w239] -> w238
                    stop <- w240 stop-if-true
                    n123 = global read "GlobalVariables.vi" "Power Meter"() -> (w239:dbl)
                    n124 = global read "GlobalVariables.vi" "Power Meter Ready"() -> (w240:bool)
                  }
                  "Power Meter" <- w238
                  n125 = local write "Power Meter"(w238) -> ()
                }
                frame #1 {
                  w242 = u16 0 items=["Full step", "Half step", "1/4 step", "1/8 step", "1/16 step", "1/32 step"] ("Step resolution")
                  # "mover motor"
                  n126 = call "RD_StepMotor_WP.vi"("Step resolution"=w242, "Direction"=TRUE, "Time between steps (ms)"=1, "Steps"=i64 1) -> ()  [unwired: 8 in]
                }
              }
              n127 = Wait (ms)(milliseconds to wait=u32 5) -> ()  [unwired: 1 out]
              n128 = feedback #1() -> (w237:dbl[])
              n129 = Build Array (concatenate)(w237, w217) -> (w212:dbl[])
              "appended array" <- w212
              n130 = Array Max & Min(array=w212) -> (max value=w214:dbl, min value=w213:dbl)  [unwired: 2 out]
              "Max Power" <- w214
              "Min Power" <- w213
              "Min Power" <- w213
              "Max Power" <- w214
              n131 = Subtract(x=w214, y=w213) -> (x-y=w230:dbl)
              n132 = Divide(x=w230, y=2.0) -> (x/y=w228:dbl)
              n133 = Add(x=w228, y=w213) -> (x+y=w231:dbl)
              n134 = call <vilib>:"Peak Detector.vi"("peaks/valleys"=enum32{"Peaks", "Valleys"}."Valleys", "width"=10 ("width 2"), "threshold"=w231, "X"=w212) -> ("Amplitudes"=→"Amplitudes":dbl[], "Locations"=w211:dbl[], "# found"=w201:i32)  [unwired: 3 in, 2 out]
              "# found" <- w201
              "Locations" <- w211
              n135 = feedback-in #1(w212) -> ()
              n136 = Equal?(x=w201, y=3) -> (x = y?=w226:bool)
              n137 = Decrement(x=w201) -> (x-1=w234:i32)
              n138 = Decrement(x=w201) -> (x-1=w199:i32)
              n139 = for {
                N: w234 -> [_]
                tunnel: w211 -> [w251]
                tunnel: [w247] -> w233 mode=indexing
                tunnel: [w246] -> w222
                i -> [w249]
                n140 = Increment(x=w249) -> (x+1=w250:i32)
                n141 = Index Array(array=w251, index #1=w250, index #2=w249) -> (element #1=w246:dbl, element #2=w248:dbl)
                n142 = Subtract(x=w246, y=w248) -> (x-y=w247:dbl)
              }
              "Array" <- w233
              n143 = Decrement(x=w199) -> (x-1=w200:i32)
              n144 = Index Array(array=w211, index=w200) -> (element=w208:dbl)
              n145 = Index Array(array=w211, index #1=w199, index #2=w200) -> (element #1=w209:dbl, element #2=w210:dbl)
              n146 = Subtract(x=w209, y=w210) -> (x-y=w205:dbl)
              n147 = Add(x=w208, y=0.0) -> (x+y=w207:dbl)
              n148 = Divide(x=w205, y=2.0) -> (x/y=w206:dbl)
              n149 = Array Subset(array=w212, index=w207, length=w206) -> (w198:dbl[])
              "Waveform Graph 2" <- w198
              n150 = Subtract(x=w223, y=w222) -> (x-y=w215:dbl)
              "step error" <- w215
              n151 = call <vilib>:"Std Deviation and Variance.vi"("X"=w233) -> ("mean"=w220:dbl, "standard deviation"=→"standard deviation":dbl)  [unwired: 1 in, 1 out]
              "mean" <- w220
              n152 = Divide(x=w220, y=2.0) -> (x/y=w219:dbl)
              n153 = global write "GlobalVariables.vi" "Power steps curve"(w198) -> ()
              n154 = To Unsigned Long Integer(number=w219) -> (unsigned 32bit integer=w218:u32)
              n155 = Array Size(array=w198) -> (size(s)=→"size(s)":i32)
              n156 = global write "GlobalVariables.vi" "Step error"(w215) -> ()
              n157 = global write "GlobalVariables.vi" "Motor Steps Max"(w218) -> ()
              "Numeric Control" <- w223
            }
          }
          frame "Get Power" {
            n158 = disable-structure shown="Enabled" {
              frame Disabled {
                n159 = call "PoweMeter-Demo.vi"("reset"=TRUE) -> ()  [unwired: 9 in, 2 out]
              }
              frame Enabled {
              }
            }
            n160 = flat-sequence {
              frame #0 {
                n161 = while {
                  stop <- w253 stop-if-true
                  n162 = global read "GlobalVariables.vi" "Power Meter"() -> (→"Power Meter":dbl)
                  n163 = global read "GlobalVariables.vi" "Power Meter Ready"() -> (w253:bool)
                }
              }
              frame #1 {
                n164 = global write "GlobalVariables.vi" "Power Meter Ready"(FALSE ("Power Meter Ready")) -> ()
              }
            }
          }
          frame "MoveMotor" {
            n165 = global read "GlobalVariables.vi" "Motor Position"() -> (w263:i32)
            n166 = global read "GlobalVariables.vi" "Motor Target"() -> (w262:dbl)
            n167 = global read "GlobalVariables.vi" "Motor Steps Max"() -> (w261:i32)
            n168 = Add(x=w263, y=w262) -> (x+y=w259:dbl)
            n169 = Increment(x=w261) -> (x+1=w257:i32)
            n170 = Greater?(x=w262, y=0.0) -> (0:w265:bool)
            n171 = Absolute Value(x=w262) -> (abs(x)=w266:dbl)
            n172 = In Range and Coerce(upper limit=w257, x=w259, lower limit=0) -> (In Range?=w258:bool)  [unwired: 1 out]
            n173 = case shown="True" w258 {
              tunnel: w266 -> [_ w272]
              tunnel: w265 -> [_ w271]
              tunnel: w259 -> [_ w268]
              frame False {
              }
              frame True {
                w270 = u16 0 items=["Full step", "Half step", "1/4 step", "1/8 step", "1/16 step", "1/32 step"] ("Step resolution")
                # "Atualiza posição Motor"
                # "LOOP de Mover o Motor"
                n174 = call "RD_StepMotor_WP.vi"("Step resolution"=w270, "Direction"=w271, "Time between steps (ms)"=10, "Steps"=w272) -> ()  [unwired: 8 in]
                n175 = global write "GlobalVariables.vi" "Motor Position"(w268) -> ()
                n176 = global write "GlobalVariables.vi" "Current Step"(w268) -> ()
                "Motor Target" <- w268
              }
            }
          }
          frame "corrects step" {
            w276 = u16 0 items=["Full step", "Half step", "1/4 step", "1/8 step", "1/16 step", "1/32 step"] ("Step resolution")
            n177 = global read "GlobalVariables.vi" "Step error"() -> (w275:i32)
            n178 = global write "GlobalVariables.vi" "Motor Position"(0 ("Current Step")) -> ()
            n179 = call "RD_StepMotor_WP.vi"("Step resolution"=w276, "Direction"=FALSE, "Time between steps (ms)"=10, "Steps"=w275) -> ()  [unwired: 8 in]
          }
        }
      }
      n180 = while {
        tunnel: w46 -> [w70]
        tunnel: w45 -> [w69]
        shift-right: [w62] -> _
        shift-left: dbl[][] [] -> [w67]
        shift-right: [w57] -> _
        shift-left: w43 -> [w58]
        shift-right: [w55] -> _
        shift-left: w43 -> [w56]
        shift-right: [w53] -> _
        shift-left: w43 -> [w54]
        shift-right: [w51] -> _
        shift-left: dbl[] [] -> [w52]
        stop <- FALSE stop-if-true
        # "Graph Loop"
        n181 = Dequeue Element(queue=w70, error in (no error)=w69) -> (element=w66:T6, error out=w68:errorcluster)  [unwired: 1 in, 2 out]
        n182 = Unbundle By Name(w66) -> ("Integration"=w61:dbl[], "Locations"=w60:dbl[], "Amplitudes"=w59:dbl[], "Signal State"=w65:string, "Step"=w63:dbl, "Spectrum"=w64:dbl[][])
        n183 = case shown="\"add spectrum\"" w65 {
          tunnel: w68 -> [_ _ _]
          tunnel: w67 -> [w96 w117 w153]
          tunnel: w64 -> [w99 _ _]
          tunnel: w63 -> [_ _ _]
          tunnel: [w95 w117 w153] -> w62
          tunnel: w61 -> [w93 _ _]
          tunnel: w60 -> [w92 _ _]
          tunnel: w59 -> [w91 _ _]
          tunnel: w58 -> [w90 w111 w152]
          tunnel: [w89 w111 w152] -> w57
          tunnel: w56 -> [w88 w110 w151]
          tunnel: [w87 w110 w151] -> w55
          tunnel: w54 -> [w86 w109 w150]
          tunnel: [w80 w109 w150] -> w53
          tunnel: w52 -> [w84 w108 w149]
          tunnel: [w77 w108 w149] -> w51
          frame "add spectrum" {
            # "Spectrum"
            # "Power"
            # "Amplitude"
            # "Location"
            # "Integration"
            n184 = global read "GlobalVariables.vi" "Current Step"() -> (w100:i32)
            n185 = global read "GlobalVariables.vi" "Step Stop"() -> (w83:i32)
            n186 = global read "GlobalVariables.vi" "Power Meter"() -> (w85:dbl)
            n187 = Index Array(array=w99, index (row) #1=0 ("index (row)"), index (row) #2=1 ("index (row)")) -> (element #2=w97:dbl[])  [unwired: 2 in, 1 out]
            n188 = Increment(x=w100) -> (x+1=w81:i32)
            n189 = Greater?(x=w81, y=w83) -> (0:w82:bool)
            n190 = global write "GlobalVariables.vi" "Motor Position"(w81) -> ()
            n191 = global write "GlobalVariables.vi" "Current Step"(w81) -> ()
            n192 = Build Array (concatenate)(w96, w97) -> (w95:dbl[][])
            "Spectrum" <- w95
            n193 = Build Array (concatenate)(w84, w85) -> (w75:dbl[])
            "Power Meter" <- w75
            n194 = Build Array (concatenate)(w90, w93) -> (w89:dbl[][])
            "Integration" <- w89
            n195 = Build Array (concatenate)(w88, w92) -> (w87:dbl[][])
            "Locations Peaks" <- w87
            n196 = Build Array (concatenate)(w86, w91) -> (w80:dbl[][])
            "Amplitudes" <- w80
            n197 = case shown="True" w82 {
              frame False {
              }
              frame True {
                n198 = global write "GlobalVariables.vi" "Experiment Running"(FALSE ("Experiment Running")) -> ()
              }
            }
            n199 = flat-sequence {
              tunnel: w75 -> [w105]
              tunnel: [w105] -> w77
              frame #0 {
                w102 = u16 0 items=["Full step", "Half step", "1/4 step", "1/8 step", "1/16 step", "1/32 step"] ("Step resolution")
                n200 = call "RD_StepMotor_WP.vi"("Step resolution"=w102, "Direction"=TRUE, "Time between steps (ms)"=1, "Steps"=i64 1) -> ()  [unwired: 8 in]
              }
            }
            n201 = Index Array(array=w80, index (col) #1=0 ("index (row)"), index (col) #2=1 ("index (row)")) -> (element #1=w79:dbl[], element #2=w74:dbl[])  [unwired: 2 in]
            n202 = Bundle(w75, w79) -> (→"Laser":cluster{dbl[], dbl[]})  [unwired: 1 in]
            n203 = Bundle(w75, w74) -> (→"Amostra":cluster{dbl[], dbl[]})  [unwired: 1 in]
          }
          frame "Save" {
            # "Spectrum"
            # "Power"
            # "Amplitude"
            # "Location"
            # "Integration"
            n204 = call <vilib>:"Application Directory.vi"() -> ("Application Directory"=w121:path)
            n205 = Build Path(base path=w121, name or relative path="Data" ("prompt (Create Folder)")) -> (appended path=w120:path)
            n206 = global read "GlobalVariables.vi" "Wavelenght"() -> (w119:dbl[])
            n207 = Insert Into Array(array=w111, index (col)=2 ("disabled index (col)"), new element=w110) -> (w115:dbl[][])  [unwired: 1 in]
            n208 = Insert Into Array(array=w115, index (col)=4 ("disabled index (col)"), new element=w109) -> (w112:dbl[][])  [unwired: 1 in]
            n209 = Insert Into Array(array=w112, index (col)=6, new element=w108) -> (w107:dbl[][])  [unwired: 1 in]
            n210 = Build Array (concatenate)(w119, w117) -> (w118:dbl[][])
            n211 = stacked-sequence {
              tunnel: w120 -> [w128 w137]
              tunnel: w118 -> [w123 _]
              tunnel: w107 -> [_ w136]
              frame #0 {
                n212 = call "Create Date Time String.vi"() -> ("Date/Time String"=w126:string)  [unwired: 10 in, 1 out]
                n213 = Concatenate Strings("Spectrum Data" ("string"), w126, ".txt" ("string")) -> (w124:string)
                n214 = Build Path(base path=w128, name or relative path=w124) -> (appended path=w132:path)
                n215 = Open/Create/Replace File(file path (use dialog)=w132, operation (0:open)=T5."replace or create", access (0:read/write)=enum16{"read/write", "read-only", "write-only"}."write-only") -> (refnum out=w135:refnum<file>)  [unwired: 3 in, 2 out]
                n216 = Refnum to Path(1:w135) -> (0:w134:path)
                n217 = call-poly <vilib>:"Write To Spreadsheet File.vi"("transpose? (no:F)"=TRUE, "format (%.3f)"="%6f" ("format string"), "2D data"=w123, "file path (dialog if empty)"=w134) -> ()  [unwired: 4 in, 1 out]
              }
              frame #1 {
                n218 = call "Create Date Time String.vi"() -> ("Date/Time String"=w140:string)  [unwired: 10 in, 1 out]
                n219 = Concatenate Strings("Peak-Integration Data" ("string"), w140, ".txt" ("string")) -> (w138:string)
                n220 = Build Path(base path=w137, name or relative path=w138) -> (appended path=w145:path)
                n221 = Open/Create/Replace File(file path (use dialog)=w145, operation (0:open)=T5."replace or create", access (0:read/write)=enum16{"read/write", "read-only", "write-only"}."write-only") -> (refnum out=w148:refnum<file>)  [unwired: 3 in, 2 out]
                n222 = Refnum to Path(1:w148) -> (0:w147:path)
                n223 = call-poly <vilib>:"Write To Spreadsheet File.vi"("transpose? (no:F)"=FALSE, "format (%.3f)"="%6f" ("format string"), "2D data"=w136, "file path (dialog if empty)"=w147) -> ()  [unwired: 4 in, 1 out]
              }
            }
          }
          frame "Reload Settings", Default {
          }
        }
      }
      n224 = Release Queue(queue=w40, error in (no error)=w39) -> (error out=w41:errorcluster)  [unwired: 1 in, 2 out]
      n225 = call <vilib>:"Simple Error Handler.vi"("error in (no error)"=w41) -> ()  [unwired: 4 in, 5 out]
    }
    frame Error {
    }
  }
  n226 = while {
    tunnel: w5 -> [w434]
    tunnel: w4 -> [_]
    tunnel: [w433] -> w11
    stop <- FALSE stop-if-true
    # "Ocean Optics"
    n227 = flat-sequence {
      tunnel: "Average" -> [w437]
      tunnel: "Integration Time" -> [w438]
      tunnel: w434 -> [w439]
      tunnel: "Correct Electrical Dark" -> [w440]
      tunnel: [w440] -> w429
      tunnel: [w439] -> w428
      tunnel: [w438] -> w427
      tunnel: [w437] -> w426
      tunnel: [w436] -> w423
      tunnel: [w446] -> w430
      tunnel: w429 -> [w449]
      tunnel: w428 -> [w447]
      tunnel: w427 -> [w445]
      tunnel: w426 -> [w444]
      tunnel: w423 -> [w441]
      tunnel: [w441] -> w422
      tunnel: [w453] -> w433
      tunnel: w430 -> [w453]
      tunnel: [w451] -> w424
      tunnel: w422 -> [w450]
      tunnel: [w450] -> w421
      frame #0 {
        n228 = Tick Count (ms)() -> (millisecond timer value=w436:u32)
      }
      frame #1 {
        n229 = call "Omni-Driver-Fast-Acquire-AVG.vi"("Average"=w444, "Correct Electrical Dark"=w449, "Spectrometer number"=0, "Integration Time (ms)"=w445, "Wrapper"=w447) -> ("Spectrum Values"=w442:dbl[], "WL Values"=w443:dbl[], "Wrapper Out"=w446:u32)  [unwired: 1 out]
        n230 = global write "GlobalVariables.vi" "Wavelenght"(w443) -> ()
        n231 = global write "GlobalVariables.vi" "Spectrum Values"(w442) -> ()
      }
      frame #2 {
        n232 = global write "GlobalVariables.vi" "Spectrum Ready"(TRUE ("Spectrum Ready")) -> ()
        n233 = Tick Count (ms)() -> (millisecond timer value=w451:u32)
      }
    }
    n234 = Subtract(x=w424, y=w421) -> (x-y=→"Spectrum delay (ms)":u32)
    n235 = Wait (ms)(milliseconds to wait=u32 10) -> ()  [unwired: 1 out]
  }
  n236 = while {
    tunnel: w2 -> [w467]
    tunnel: w1 -> [w461]
    tunnel: [w468] -> w14
    tunnel: [w458] -> w13
    stop <- "Stop" stop-if-true
    # "Get Power"
    # "Power Meter"
    n237 = flat-sequence {
      tunnel: w461 -> [w473]
      tunnel: [w473] -> w460
      tunnel: [w472] -> w456
      frame #0 {
        n238 = Tick Count (ms)() -> (millisecond timer value=w472:u32)
      }
    }
    n239 = Wait (ms)(milliseconds to wait=u32 10) -> ()  [unwired: 1 out]
    n240 = call "TLPM Set Average Time.vi"("error in (no error)"=w460, "Average Time (0.0)"="Average Time (0.0)", "instrument handle"=w467) -> ("error out"=w465:errorcluster, "instrument handle out"=w469:refnum<visa-resource-name>)  [unwired: 7 in]
    n241 = call "TLPM Measure Power.vi"("error in (no error)"=w465, "instrument handle"=w469) -> ("error out"=w462:errorcluster, "Power"=w463:dbl, "instrument handle out"=w468:refnum<visa-resource-name>)  [unwired: 7 in]
    "Power Value" <- w463
    n242 = global write "GlobalVariables.vi" "Power Meter"(w463) -> ()
    n243 = flat-sequence {
      tunnel: w462 -> [w475]
      tunnel: [w475] -> w459
      frame #0 {
        n244 = global write "GlobalVariables.vi" "Power Meter Ready"(TRUE ("Power Meter Ready")) -> ()
      }
    }
    n245 = flat-sequence {
      tunnel: w459 -> [w471]
      tunnel: [w471] -> w458
      tunnel: [w470] -> w457
      frame #0 {
        n246 = Tick Count (ms)() -> (millisecond timer value=w470:u32)
      }
    }
    n247 = Subtract(x=w457, y=w456) -> (x-y=→"P Meter Delay (ms)":u32)
  }
  n248 = call "Omni-Driver-Fast-Close.vi"("Wrapper In"=w11) -> ()  [unwired: 1 in]
  n249 = call "TLPM Close.vi"("error in (no error)"=w13, "instrument handle"=w14) -> ("error out"=w12:errorcluster)  [unwired: 9 in]
  n250 = flat-sequence {
    tunnel: w12 -> [_]
    frame #0 {
      n251 = Stop() -> ()  [unwired: 1 in]
    }
  }
